vi "5302Unformat.vi"(11 "Data String":string) -> (2 "Numeric 2":i32, 3 "Numeric 1":i32)   [LabVIEW 2015]
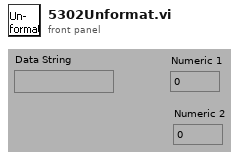
[diagram p1: front panel]
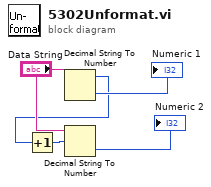
[diagram p0: block diagram]
diagram:
  n1 = Decimal String To Number(string="Data String") -> (offset past number=w3:i32, number=→"Numeric 1":i32)  [unwired: 2 out]
  n2 = Increment(x=w3) -> (x+1=w1:i32)
  n3 = Decimal String To Number(string="Data String", offset=w1) -> (number=→"Numeric 2":i32)  [unwired: 2 out]
